vi "Keithley 6430 Read.vi"(2 "Point #":i32, 3 "Instrument Address":refnum<visa-resource-name>) -> (0 "Stop":bool, 1 "Measurement":dbl[](array[numeric]) format="%.6e")   [LabVIEW 2020]
doc: "This VI reads a single reading from a Keithley 2001 multimeter. The stop boolean is always false. If no reading is obtained a single zero is returned.\nScott Hannahs, NHMFL-FSU, Nov 1993"
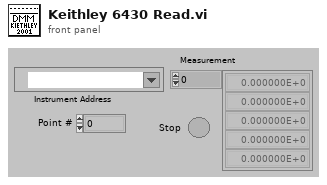
[diagram p1: front panel]
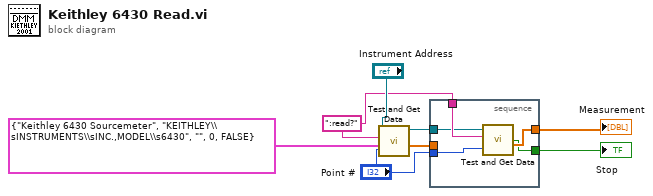
[diagram p0: block diagram]
diagram:
  w4 = ":read?"
  n1 = call "Test and Get Data.vi"("Point #"="Point #", "Instrument Info"=cluster{string, string, string, u32, bool} {"Keithley 6430 Sourcemeter", "KEITHLEY\\sINSTRUMENTS\\sINC.,MODEL\\s6430", "", 0, FALSE}, "Command String"=w4, "VISA Sesson"="Instrument Address") -> ("Measurement"=w2:dbl[], "dup VISA session"=w1:refnum<visa-resource-name>)  [unwired: 2 in, 3 out]
  n2 = stacked-sequence {
    tunnel: [w13] -> w7
    tunnel: [w12] -> w6
    tunnel: w4 -> [w11]
    tunnel: "Point #" -> [w10]
    tunnel: w2 -> [_]
    tunnel: w1 -> [w9]
    frame #0 {
      n3 = call "Test and Get Data.vi"("Point #"=w10, "Command String"=w11, "VISA Sesson"=w9) -> ("Measurement"=w13:dbl[], "Stop"=w12:bool)  [unwired: 3 in, 3 out]
    }
  }
  "Stop" <- w6
  "Measurement" <- w7
